vi "NT Write Value.vi"   [LabVIEW 2025]
doc: "A polymorphic VI that will write the data to the named entry. It adapts to the data type you wire to it."
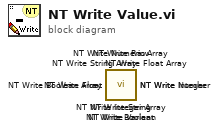
[diagram p0: block diagram]
diagram:
  n1 = call <vilib>:"NT Write Integer Array.vi"() -> ()  [unwired: 11 in, 1 out]
  n2 = call <vilib>:"NT Write Float Array.vi"() -> ()  [unwired: 11 in, 1 out]
  n3 = call <vilib>:"NT Write Float.vi"() -> ()  [unwired: 11 in, 1 out]
  n4 = call <vilib>:"NT Write Integer.vi"() -> ()  [unwired: 11 in, 1 out]
  n5 = call <vilib>:"NT Write Variant.vi"() -> ()  [unwired: 11 in, 1 out]
  n6 = call <vilib>:"NT Write Raw.vi"() -> ()  [unwired: 11 in, 1 out]
  n7 = call <vilib>:"NT Write String Array.vi"() -> ()  [unwired: 11 in, 1 out]
  n8 = call <vilib>:"NT Write Numeric Array.vi"() -> ()  [unwired: 11 in, 1 out]
  n9 = call <vilib>:"NT Write Boolean Array.vi"() -> ()  [unwired: 11 in, 1 out]
  n10 = call <vilib>:"NT Write String.vi"() -> ()  [unwired: 11 in, 1 out]
  n11 = call <vilib>:"NT Write Number.vi"() -> ()  [unwired: 11 in, 1 out]
  n12 = call <vilib>:"NT Write Boolean.vi"() -> ()  [unwired: 11 in, 1 out]
